vi "Visual_sorting_ABB_ByLabview.vi"() -> ()   [LabVIEW 2016]
panel:
  in  "停止按钮":bool
  in  "停止":bool
  out "send to robot":string
  out "耗时":u32=175
  out "Calibrated Image 2":T1(plugin-control)
  out "红色":i32[](array[numeric])=[0, 0, 1]
  out "耗时":u32=11084218
  # "蓝色"
  # "黑色"
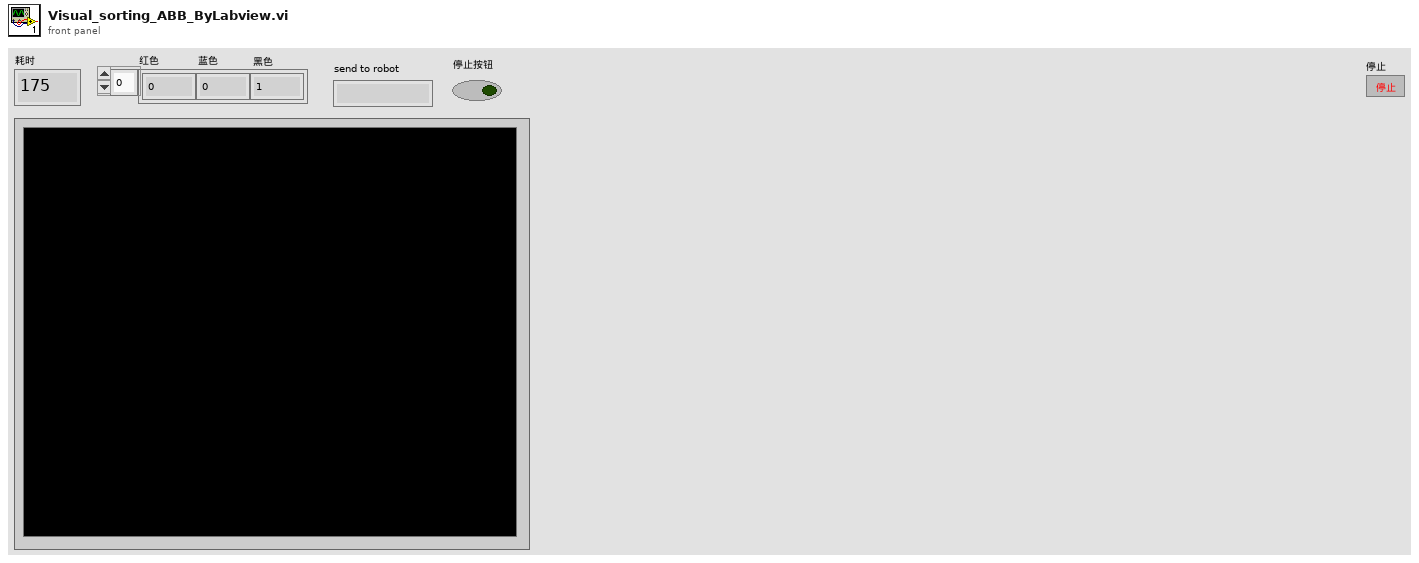
[diagram p1: front panel]
types:
  T1 = typedef "IMAQ Image.ctl" = refnum<image>
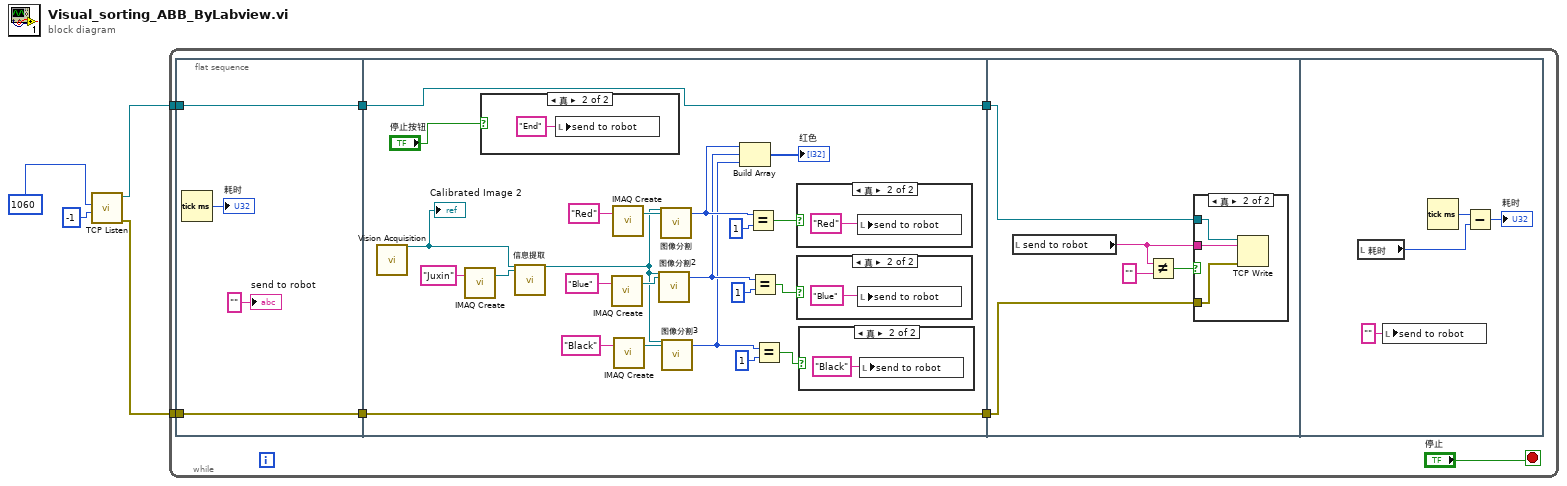
[diagram p0: block diagram]
diagram:
  n1 = call <vilib>:"TCP Listen.vi"("timeout ms (wait forever: -1)"=-1, "port"=u16 1060) -> ("error out"=w2:errorcluster, "connection ID"=w3:refnum<k5>)  [unwired: 5 in, 3 out]
  n2 = while {
    tunnel: w3 -> [w10]
    tunnel: w2 -> [w9]
    stop <- "停止" stop-if-true
    n3 = flat-sequence {
      tunnel: w10 -> [w13]
      tunnel: [w13] -> w11
      tunnel: w9 -> [w12]
      tunnel: [w12] -> w8
      tunnel: w11 -> [w18]
      tunnel: [w18] -> w7
      tunnel: [w17] -> w6
      tunnel: w8 -> [w17]
      tunnel: w7 -> [w45]
      tunnel: w6 -> [w43]
      frame #0 {
        n4 = Tick Count (ms)() -> (millisecond timer value=→"耗时":u32)
        "send to robot" <- "" ("send to robot")
      }
      frame #1 {
        n5 = call "Vision Acquisition"() -> ("Image Out"=w22:T1)  [unwired: 23 in, 4 out]
        "Calibrated Image 2" <- w22
        n6 = call "IMAQ Create"("Image Name"="Juxin") -> ("New Image"=w38:T1)  [unwired: 4 in, 1 out]
        n7 = case shown="真" "停止按钮" {
          frame False {
          }
          frame True {
            n8 = local write "send to robot"("End" ("send to robot")) -> ()
          }
        }
        n9 = call "信息提取"("Image In"=w22, "Image Dst"=w38) -> ("Image Out"=w30:T1)  [unwired: 24 in, 1 out]
        n10 = call "IMAQ Create"("Image Name"="Blue") -> ("New Image"=w33:T1)  [unwired: 4 in, 1 out]
        n11 = call "IMAQ Create"("Image Name"="Red") -> ("New Image"=w35:T1)  [unwired: 4 in, 1 out]
        n12 = call "IMAQ Create"("Image Name"="Black") -> ("New Image"=w32:T1)  [unwired: 4 in, 1 out]
        n13 = call "图像分割2"("Image In"=w30, "Image Dst"=w33) -> ("Number of Particles (Particle Analysis 1)"=w25:i32)  [unwired: 23 in, 2 out]
        n14 = call "图像分割"("Image In"=w30, "Image Dst"=w35) -> ("Number of Particles (Particle Analysis 1)"=w26:i32)  [unwired: 23 in, 2 out]
        n15 = call "图像分割3"("Image In"=w30, "Image Dst"=w32) -> ("Number of Particles (Particle Analysis 1)"=w24:i32)  [unwired: 23 in, 2 out]
        n16 = Build Array(w26, w25, w24) -> (→"红色":i32[])
        n17 = Equal?(x=w26, y=1) -> (x = y?=w21:bool)
        n18 = Equal?(x=w25, y=1) -> (x = y?=w20:bool)
        n19 = Equal?(x=w24, y=1) -> (x = y?=w19:bool)
        n20 = case shown="真" w21 {
          frame False {
          }
          frame True {
            n21 = local write "send to robot"("Red") -> ()
          }
        }
        n22 = case shown="真" w20 {
          frame False {
          }
          frame True {
            n23 = local write "send to robot"("Blue") -> ()
          }
        }
        n24 = case shown="真" w19 {
          frame False {
          }
          frame True {
            n25 = local write "send to robot"("Black") -> ()
          }
        }
      }
      frame #2 {
        n26 = local read "send to robot"() -> (w44:string)
        n27 = Not Equal?(x=w44, y="" ("send to robot")) -> (x != y?=w46:bool)
        n28 = case shown="真" w46 {
          tunnel: w45 -> [_ w50]
          tunnel: w44 -> [_ w49]
          tunnel: w43 -> [_ w48]
          frame False {
          }
          frame True {
            n29 = TCP Write(connection ID=w50, data in=w49, error in (no error)=w48) -> ()  [unwired: 1 in, 3 out]
          }
        }
      }
      frame #3 {
        n30 = local read "耗时"() -> (w53:u32)
        n31 = local write "send to robot"("" ("send to robot")) -> ()
        n32 = Tick Count (ms)() -> (millisecond timer value=w54:u32)
        n33 = Subtract(x=w54, y=w53) -> (x-y=→"耗时":u32)
      }
    }
  }
